vi "XYZ Move.vi"(6 "Wait For Motion Done?":bool, 8 "error in (no error)":errorcluster, 9 "Motion Mode":enum16{"Absolute", "Relative"}(ring), 10 "Destination [mm]":dbl[](array[numeric]), 11 "LSID":i32) -> (0 "error out":errorcluster)   [LabVIEW 2014]
uses:
  <userlib>/Tango_DLL/Tango_DLL.lvlib
panel:
  # "LICENSED MATERIALS – PROPERTY OF IBM\nCopyright IBM Corp. 2016,\nALL RIGHTS RESERVED"
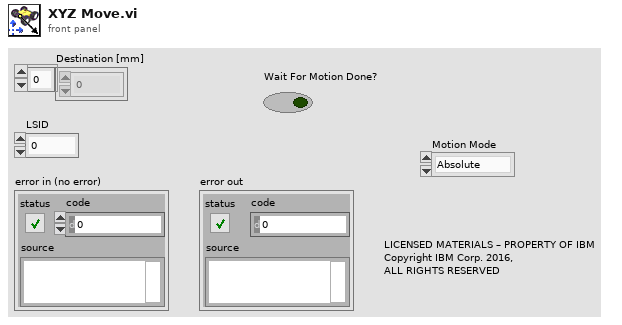
[diagram p1: front panel]
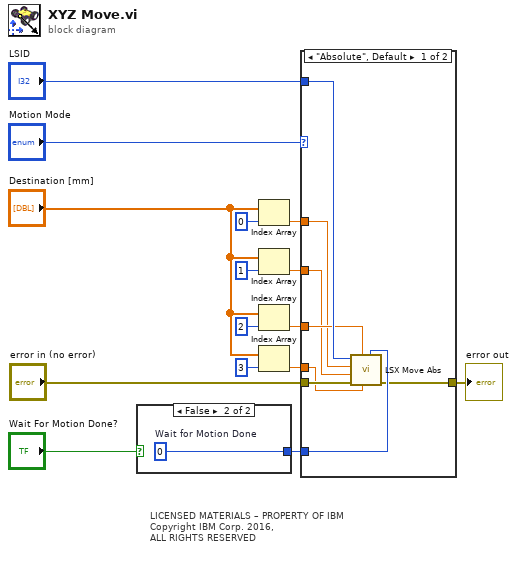
[diagram p0: block diagram]
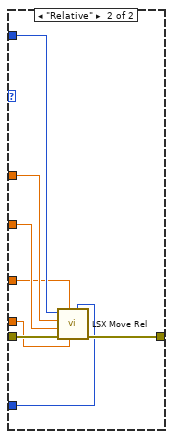
[diagram p2: hidden frame]
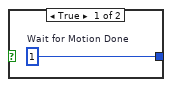
[diagram p3: hidden frame]
diagram:
  # "LICENSED MATERIALS – PROPERTY OF IBM\nCopyright IBM Corp. 2016,\nALL RIGHTS RESERVED"
  n1 = case shown="False" "Wait For Motion Done?" {
    tunnel: [w16 w17] -> w15
    frame True {
      w16 = 1  # Wait for Motion Done
    }
    frame False, Default {
      w17 = 0  # Wait for Motion Done
    }
  }
  n2 = Index Array(array="Destination [mm]", index=0) -> (element=w3:dbl)
  n3 = Index Array(array="Destination [mm]", index=1) -> (element=w4:dbl)
  n4 = Index Array(array="Destination [mm]", index=2) -> (element=w5:dbl)
  n5 = Index Array(array="Destination [mm]", index=3) -> (element=w6:dbl)
  n6 = case shown="\"Absolute\", Default" "Motion Mode" {
    tunnel: w15 -> [w25 w26]
    tunnel: "error in (no error)" -> [w24 w33]
    tunnel: [w23 w32] -> w12
    tunnel: "LSID" -> [w22 w31]
    tunnel: w6 -> [w21 w27]
    tunnel: w5 -> [w20 w28]
    tunnel: w4 -> [w19 w29]
    tunnel: w3 -> [w18 w30]
    frame "Absolute", Default {
      n7 = call <userlib>:"LSX Move Abs.vi"("bWait"=w25, "dA"=w21, "dZ"=w20, "error in (no error)"=w24, "dY"=w19, "dX"=w18, "lLSID"=w22) -> ("error out"=w23:errorcluster)  [unwired: 3 in, 1 out]
    }
    frame "Relative" {
      n8 = call <userlib>:"LSX Move Rel.vi"("bWait"=w26, "dA"=w27, "dZ"=w28, "error in (no error)"=w33, "dY"=w29, "dX"=w30, "lLSID"=w31) -> ("error out"=w32:errorcluster)  [unwired: 3 in, 1 out]
    }
  }
  "error out" <- w12
